vi "Find_Unique_Filename.vi"(0 "Path In":path, 1 "Max Length (31)":i32=31) -> (3 "Unique Path Out":path)   [LabVIEW 2018]
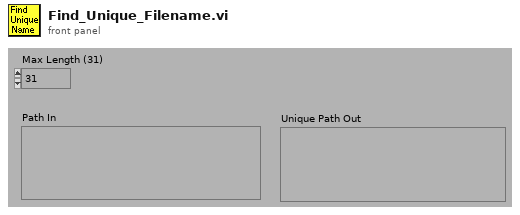
[diagram p1: front panel]
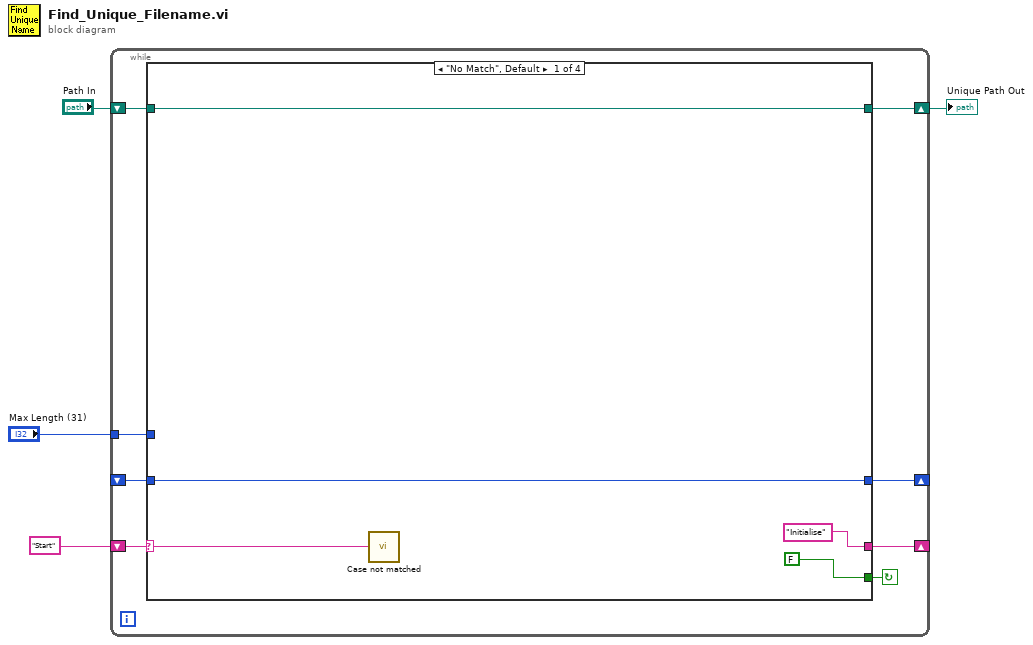
[diagram p0: block diagram]
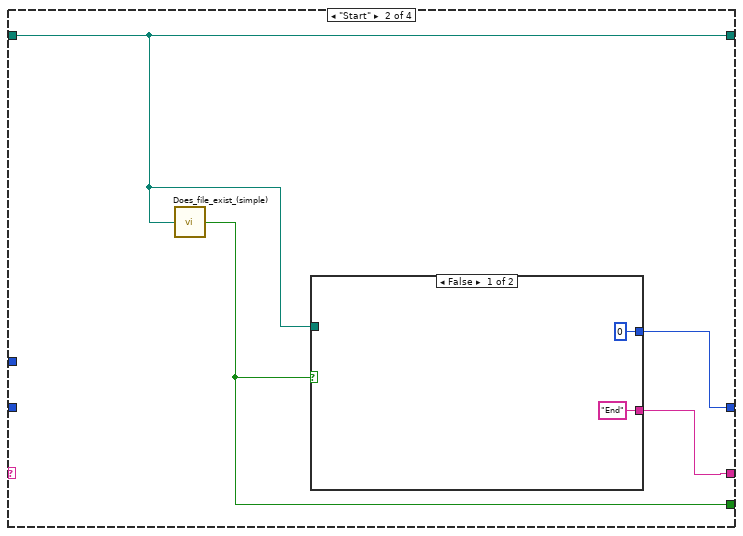
[diagram p2: hidden frame]
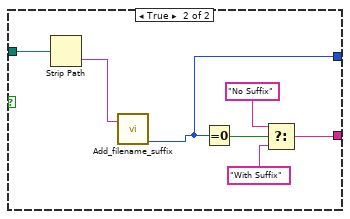
[diagram p3: hidden frame]
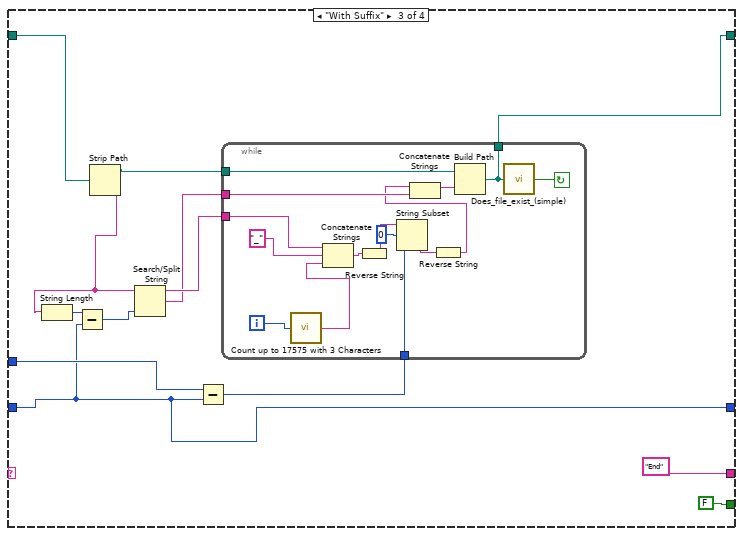
[diagram p4: hidden frame]
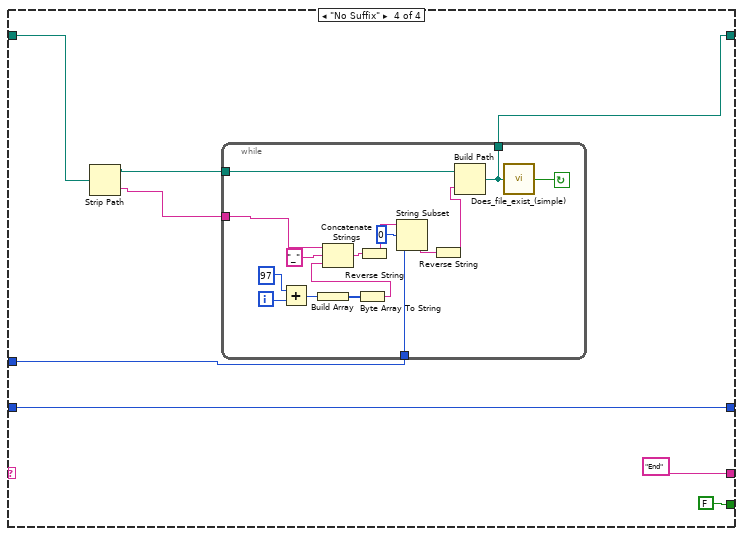
[diagram p5: hidden frame]
diagram:
  n1 = while {
    shift-left: "Start" -> [w10]
    shift-right: [w11] -> _
    shift-right: [w8] -> w2
    shift-left: "Path In" -> [w9]
    tunnel: "Max Length (31)" -> [w7]
    shift-right: [w6] -> _
    shift-left: _ -> [w5]
    stop <- w12 continue-if-true
    n2 = case shown="\"No Match\", Default" w10 {
      selector: w10 -> [w13 _ _ _]
      tunnel: [FALSE w20 FALSE FALSE] -> w12
      tunnel: ["Initialise" w21 "End" "End"] -> w11
      tunnel: w9 -> [w15 w19 w36 w63]
      tunnel: [w15 w19 w35 w62] -> w8
      tunnel: w7 -> [_ _ w38 w60]
      tunnel: [w14 w18 w31 w59] -> w6
      tunnel: w5 -> [w14 _ w31 w59]
      frame "No Match", Default {
        n3 = call "Case not matched.vi"("Case Name not Matched"=w13) -> ()
      }
      frame "Start" {
        n4 = call "Does_file_exist_(simple).vi"("Pathname"=w19) -> ("exists?"=w20:bool)
        n5 = case shown="False" w20 {
          tunnel: ["End" w29] -> w21
          tunnel: w19 -> [_ w26]
          tunnel: [0 ("Extension length") w24] -> w18
          frame False {
          }
          frame True {
            n6 = Strip Path(path=w26) -> (name=w25:string)  [unwired: 1 out]
            n7 = call "Add_filename_suffix.vi"("Filename"=w25) -> ("Extension length"=w24:i32)  [unwired: 1 in, 3 out]
            n8 = Equal To 0?(x=w24) -> (x = 0?=w30:bool)
            n9 = Select(t="No Suffix", s=w30, f="With Suffix") -> (s? t:f=w29:string)
          }
        }
      }
      frame "With Suffix" {
        n10 = Strip Path(path=w36) -> (stripped path=w41:path, name=w40:string)
        n11 = String Length(string=w40) -> (length=w39:i32)
        n12 = Subtract(x=w39, y=w31) -> (x-y=w34:i32)
        n13 = Search/Split String(string=w40, offset (0)=w34) -> (substring before match=w33:string, match + rest of string=w32:string)  [unwired: 2 out]
        n14 = Subtract(x=w38, y=w31) -> (x-y=w37:i32)
        n15 = while {
          tunnel: w33 -> [w58]
          tunnel: w37 -> [w57]
          tunnel: w41 -> [w56]
          tunnel: w32 -> [w55]
          tunnel: [w47] -> w35
          i -> [w45]
          stop <- w48 continue-if-true
          n16 = call "Count up to 17575 with 3 Characters.vi"("Numeric Control"=w45) -> ("string"=w44:string)
          n17 = Concatenate Strings(w58, "_" ("string"), w44) -> (w53:string)
          n18 = Reverse String(1:w53) -> (0:w54:string)
          n19 = String Subset(string=w54, offset (0)=0, length (rest)=w57) -> (substring=w52:string)
          n20 = Reverse String(1:w52) -> (0:w50:string)
          n21 = Concatenate Strings(w50, w55) -> (w49:string)
          n22 = Build Path(base path=w56, name or relative path=w49) -> (appended path=w47:path)
          n23 = call "Does_file_exist_(simple).vi"("Pathname"=w47) -> ("exists?"=w48:bool)
        }
      }
      frame "No Suffix" {
        n24 = Strip Path(path=w63) -> (stripped path=w64:path, name=w61:string)
        n25 = while {
          tunnel: w61 -> [w82]
          tunnel: w60 -> [w81]
          tunnel: w64 -> [w80]
          tunnel: [w70] -> w62
          i -> [w72]
          stop <- w71 continue-if-true
          n26 = Add(x=97, y=w72) -> (x+y=w78:i32)
          n27 = Build Array(w78) -> (w79:i32[])
          n28 = Byte Array To String(unsigned byte array=w79) -> (string=w68:string)
          n29 = Concatenate Strings(w82, "_" ("string"), w68) -> (w75:string)
          n30 = Reverse String(1:w75) -> (0:w76:string)
          n31 = String Subset(string=w76, offset (0)=0, length (rest)=w81) -> (substring=w74:string)
          n32 = Reverse String(1:w74) -> (0:w69:string)
          n33 = Build Path(base path=w80, name or relative path=w69) -> (appended path=w70:path)
          n34 = call "Does_file_exist_(simple).vi"("Pathname"=w70) -> ("exists?"=w71:bool)
        }
      }
    }
  }
  "Unique Path Out" <- w2
